vi "Create Test Configuration.vi"() -> (0 "error out":errorcluster, 1 "Names":string[](array[string]), 2 "Line Array":T1(array[cluster]), 3 "Module":refnum<class "Central Error Handler configuration.lvclass">, 4 "Channels":refnum<class "TBM channel.lvclass">[](array[class]), 5 "instance identifier":string)   [LabVIEW 2017, in "Central Error Handler tests.lvlib"]
uses:
  Central Error Handler tests.lvlib
  <vilib>/NI/Tag Bus Module Framework/channel/TBM channel.lvclass
  module/configuration/Central Error Handler configuration.lvclass
  C:/Program Files (x86)/National Instruments/LabVIEW 2017/vi.lib/NI/Configuration Framework/serializable configuration/NISE_CEF_serializable configuration.lvclass
  C:/Program Files (x86)/National Instruments/LabVIEW 2017/vi.lib/NI/DCAF/Tag Editor Core/control module/configuration/control module configuration.lvclass
  <vilib>/NI/Tag Bus Module Framework/channel/channel classification.ctl
  <vilib>/NI/Configuration Framework/serializable configuration/NISE_CEF_serializable configuration.lvclass
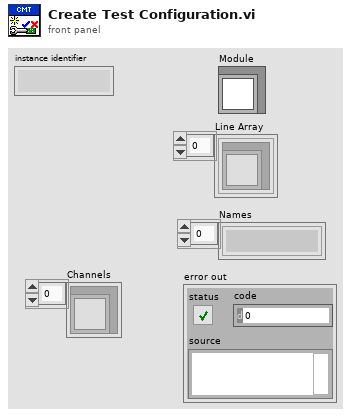
[diagram p1: front panel]
types:
  T1 = cluster{"channel":refnum<class "TBM channel.lvclass">}[]
  T2 = typedef "TBM channel.lvclass/channel classification.ctl" = enum16{"input data", "output data", "processing parameter", "processing result"}
  T3 = typedef "tag bus.lvlib/tag descriptor.lvclass/Data Type.ctl" = enum16{"Double", "Single", "I64", "I32", "I16", "I8", "U64", "U32", "U16", "U8", "Boolean", "String", "Array of Double", "Array of Single", "Array of I64", "Array of I32", "Array of I16", "Array of I8", "Array of U64", "Array of U32", "Array of U16", "Array of U8", "Array of Boolean", "Array of String"}
  T4 = cluster{"channel":refnum<class "TBM channel.lvclass">}
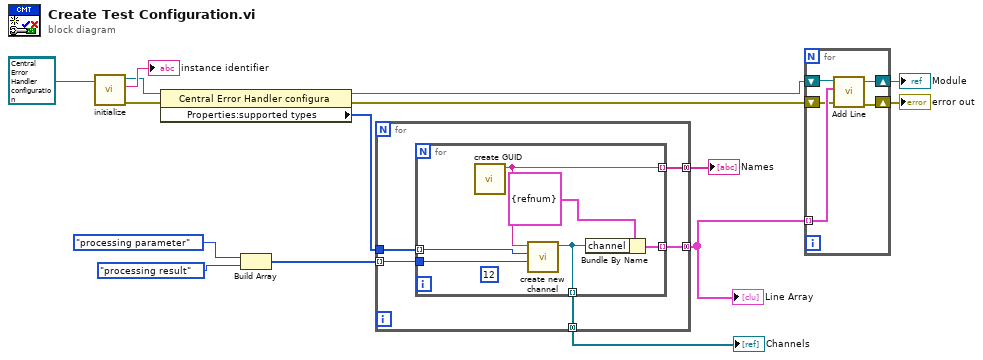
[diagram p0: block diagram]
diagram:
  (unwired) refnum<class "Central Error Handler configuration.lvclass"> refnum ("user control module configuration")
  n1 = call <vilib>:"initialize.vi"("configuration in"=refnum<class "Central Error Handler configuration.lvclass"> refnum ("user control module configuration")) -> ("error out"=w14:errorcluster, "identifier"=→"instance identifier":string, "configuration out"=w11:refnum<class "Central Error Handler configuration.lvclass">)  [unwired: 8 in]
  n2 = property class="Central Error Handler configura"(reference=w11, error in=w14) -> (reference out=w8:refnum<class "Central Error Handler configuration.lvclass">, error out=w13:errorcluster, "Properties:supported types"=w9:T3[])
  n3 = Build Array(channel_classification."processing parameter" ("channel classification"), channel_classification."processing result" ("channel classification")) -> (w7:T2[])
  n4 = for {
    tunnel: w7 -> [w20] mode=indexing
    tunnel: [w18] -> w10 mode=concatenating
    tunnel: w9 -> [w19]
    tunnel: [w17] -> w12 mode=concatenating
    tunnel: [w16] -> w4 mode=concatenating
    n5 = for {
      tunnel: w20 -> [w26]
      tunnel: [w23] -> w18 mode=indexing
      tunnel: w19 -> [w25] mode=indexing
      tunnel: [w24] -> w17 mode=indexing
      tunnel: [w22] -> w16 mode=indexing
      (unwired) 12
      n6 = call <vilib>:"create GUID.vi"() -> ("uuid"=w24:string)  [unwired: 10 in, 1 out]
      n7 = call <vilib>:"create new channel.vi"("channel classification"=w26, "data type"=w25, "channel name"=w24) -> ("channel"=w22:refnum<class "TBM channel.lvclass">)  [unwired: 8 in]
      n8 = Bundle By Name(cluster=T4 {"channel"=refnum} ("Line"), "channel"=w22) -> (w23:T4)
    }
  }
  "Names" <- w12
  "Channels" <- w4
  "Line Array" <- w10
  n9 = for {
    tunnel: w10 -> [w29] mode=indexing
    shift-right: [w30] -> w2
    shift-left: w8 -> [w31]
    shift-right: [w27] -> w1
    shift-left: w13 -> [w28]
    n10 = call-dynamic "Add Line.vi"("error in (no error)"=w28, "Line"=w29, "Central Error Handler configuration in"=w31) -> ("error out"=w27:errorcluster, "Central Error Handler configuration out"=w30:refnum<class "Central Error Handler configuration.lvclass">)  [unwired: 7 in]
  }
  "Module" <- w2
  "error out" <- w1
